vi "Write Load Control.vi"(8 "error in":errorcluster, 10 "Load_Control":T1, 11 "Load in":refnum<class "Load.lvclass">) -> (0 "error out":errorcluster, 3 "Load out":refnum<class "Load.lvclass">)   [LabVIEW 2018, in "Load Actor.lvlib" / "Load.lvclass"]
uses:
  Load.lvclass
  C:/Users/Administrator/Desktop/2018LabVIEW EMS/IED Actors/Device DDS Communications Framework/Device DDS Communications/Device DDS Communications.lvclass
  <vilib>/ORNL/CSEISMIC DDS/CSEISMIC DDS Base/Data Types/Load_Control.ctl
  <vilib>/ORNL/CSEISMIC DDS/CSEISMIC DDS Base/Data Types/Controls/DeviceID.ctl
  Device DDS Communications Framework/Device DDS Communications/Device DDS Communications.lvclass/Device DDS Communications.ctl
  <vilib>/ORNL/CSEISMIC DDS/CSEISMIC DDS Base/CSEISMIC DDS.lvclass/CSEISMIC DDS.ctl
  <vilib>/ORNL/CSEISMIC DDS/CSEISMIC DDS Base/Accessors/Read DDS Reference.vi
  <vilib>/ORNL/CSEISMIC DDS/DDS Writer/DDS Writer.lvclass
  C:/Program Files (x86)/National Instruments/LabVIEW 2018/vi.lib/ORNL/CSEISMIC DDS/CSEISMIC DDS Base/CSEISMIC DDS.lvclass
  <vilib>/ORNL/CSEISMIC DDS/CSEISMIC DDS Base/Error Handler.vi
  Device DDS Communications Framework/Device DDS Communications/Device DDS Communications.lvclass
  <vilib>/ORNL/CSEISMIC DDS/CSEISMIC DDS Base/CSEISMIC DDS.lvclass
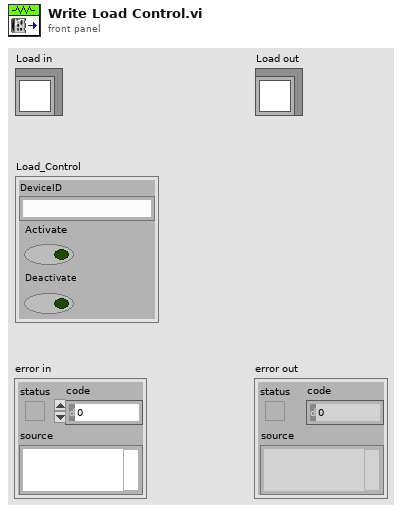
[diagram p1: front panel]
types:
  T1 = typedef "CSEISMIC DDS.lvlib/CSEISMIC DDS.lvclass/Load_Control.ctl" = cluster{"DeviceID":T2, "Activate":bool, "Deactivate":bool}
  T2 = typedef "CSEISMIC DDS.lvlib/CSEISMIC DDS.lvclass/DeviceID.ctl" = string
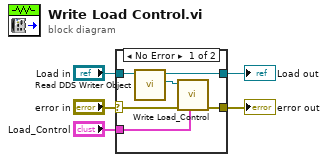
[diagram p0: block diagram]
diagram:
  n1 = case shown="No Error" "error in" {
    selector: "error in" -> [w7 w13]
    tunnel: [w8 w13] -> w4
    tunnel: [w10 w12] -> w2
    tunnel: "Load in" -> [w9 w12]
    tunnel: "Load_Control" -> [w6 _]
    frame No Error {
      n2 = call "Read DDS Writer Object.vi"("Device DDS Communications in"=w9) -> ("DDS Writer Object"=w11:refnum<class "DDS Writer.lvclass">, "Device DDS Communications out"=w10:refnum<class "Load.lvclass">)  [unwired: 9 in]
      n3 = call <vilib>:"Write Load_Control.vi"("Load_Control"=w6, "error in"=w7, "DDS Writer in"=w11) -> ("error out"=w8:errorcluster)  [unwired: 7 in, 1 out]
    }
    frame Error {
    }
  }
  "error out" <- w4
  "Load out" <- w2
